vi "Pack Channels with Interleaving Select.vi"(0 "Array":cluster{i16[]}[](array[cluster]), 1 "interleaving factor":u16, 5 "channels enabled":u64 caption="stream.num samples 0", 7 "data valid?":bool) -> (4 "Array out":cluster{i16[]}[](array[cluster]), 6 "channels enabled out":u64, 8 "data valid":bool)   [LabVIEW 2018, in "GettingStarted_5774_FPGA.lvlib"]
uses:
  GettingStarted_5774_FPGA.lvlib
  8d920cb7-4e87-4db0-a654-5043d689489d.vi
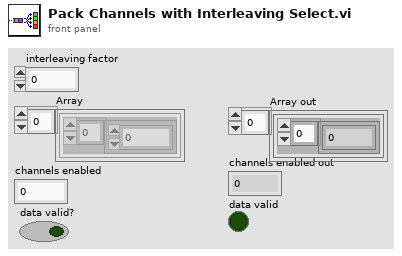
[diagram p1: front panel]
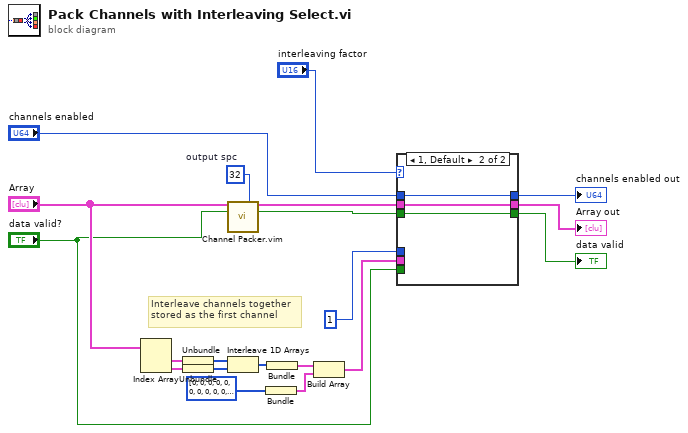
[diagram p0: block diagram]
diagram:
  w9 = 32  # output spc
  # "Interleave channels together\nstored as the first channel"
  n1 = Index Array(array="Array") -> (element #1=w17:cluster{i16[]}, element #2=w16:cluster{i16[]})  [unwired: 2 in]
  n2 = Unbundle(w17) -> (w15:i16[])
  n3 = Unbundle(w16) -> (w14:i16[])
  n4 = call "Channel Packer.vim"("Array in"="Array", "output spc"=w9, "data valid"="data valid?") -> ("Array out"=w2:cluster{i16[]}[], "full"=w1:bool)  [unwired: 11 in]
  n5 = Interleave 1D Arrays(w15, w14) -> (w13:i16[])
  n6 = Bundle(i16[] [0, 0, 0, 0, 0, 0, 0, 0, 0, 0, 0, 0, 0, 0, 0, 0, 0, 0, 0, 0, 0, 0, 0, 0, 0, 0, 0, 0, 0, 0, 0, 0]) -> (w10:cluster{i16[]})  [unwired: 1 in]
  n7 = Bundle(w13) -> (w11:cluster{i16[]})  [unwired: 1 in]
  n8 = Build Array(w11, w10) -> (w8:cluster{i16[]}[])
  n9 = case shown="1, Default" "interleaving factor" {
    tunnel: [w22 w25] -> w19
    tunnel: [w23 w24] -> w18
    tunnel: [w21 w26] -> w20
    tunnel: w8 -> [w22 _]
    tunnel: u64 1 ("flexrio.stream.channels enabled 0") -> [w21 _]
    tunnel: "data valid?" -> [w23 _]
    tunnel: "channels enabled" -> [_ w26]
    tunnel: w2 -> [_ w25]
    tunnel: w1 -> [_ w24]
    frame 2 {
    }
    frame 1, Default {
    }
  }
  "channels enabled out" <- w20
  "Array out" <- w19
  "data valid" <- w18
